vi "UPDATE_volume_by_path.vi"(8 "error in (no error)":errorcluster, 11 "volume path":path) -> (0 "error out":errorcluster)   [LabVIEW 2024]
uses:
  <vilib>/addons/_JKI.lib/Serialization/JSON/JKI JSON Serialization.lvlib
panel:
  in  "from id?":bool
  in  "id":i32
  out "json filename":string
  out "Numeric":i32
  out "appended path":path
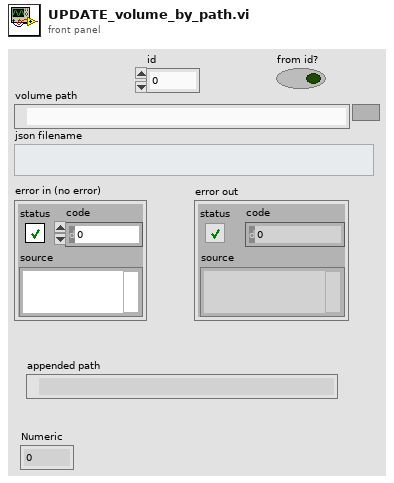
[diagram p1: front panel]
types:
  T1 = typedef "local_volume.ctl" = cluster{"id":i32, "name":string, "sortable_name":string, "aliases":string[], "description":string, "site_detail_url":string, "count_of_issues":i32, "start_year":i32, "publisher_id":i32, "issue_ids":i32[], "date_last_updated":timestamp, "volume":i32, "cv_id":string}
  T2 = typedef "local_issue.ctl" = cluster{"cover_date":timestamp, "id":i32, "cv_id":string, "name":string, "sortable_name":string, "issue_number":string, "deck":string, "description":string, "volume":T3, "store_date":timestamp, "date_last_updated":timestamp, "site_detail_url":string, "cover_url":string, "associated_images":T4[], "characters":T3[], "concepts":T3[], "creators":T5[], "storyArcs":T3[], "teams":T3[]}
  T3 = typedef "comicvine_issue.generic_credit.ctl" = cluster{"id":i32, "name":string}
  T4 = typedef "comicvine_issue.associated_image.ctl" = cluster{"original_url":string, "id":i32}
  T5 = typedef "comicvine_issue.person_credit.ctl" = cluster{"id":i32, "name":string, "role":string}
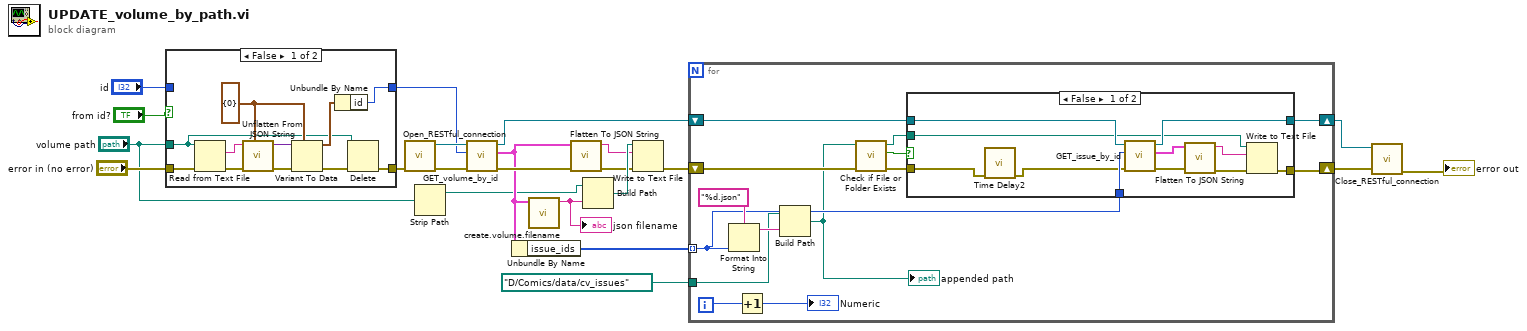
[diagram p0: block diagram]
diagram:
  n1 = case shown="False" "from id?" {
    tunnel: "error in (no error)" -> [w31 w34]
    tunnel: [w27 w34] -> w6
    tunnel: "volume path" -> [w24 _]
    tunnel: [w23 w35] -> w1
    tunnel: "id" -> [_ w35]
    frame False {
      w26 = cluster{"id":i32} {"id"=0}
      n2 = Read from Text File(file (use dialog)=w24, error in=w31) -> (text=w33:string, error out=w30:errorcluster)  [unwired: 2 in, 2 out]
      n3 = call <vilib>:"Unflatten From JSON String.vi"("Type and Defaults"=w26, "error in (no error)"=w30, "JSON String"=w33) -> ("error out"=w29:errorcluster, "Variant"=w32:variant)  [unwired: 7 in]
      n4 = Variant To Data(error in=w29, type=w26, Variant=w32) -> (data=w25:cluster{"id":i32}, error out=w28:errorcluster)
      n5 = Unbundle By Name(w25) -> ("id"=w23:i32)
      n6 = Delete(path (use dialog)=w24, error in=w28) -> (error out=w27:errorcluster)  [unwired: 3 in, 2 out]
    }
    frame True {
    }
  }
  n7 = call "Open_RESTful_connection.vi"("error in (no error)"=w6) -> ("error out"=w12:errorcluster, "REST Client out"=w22:refnum<class "REST Client.lvclass">)  [unwired: 9 in]
  n8 = Strip Path(path="volume path") -> (stripped path=w4:path)  [unwired: 1 out]
  n9 = call "GET_volume_by_id.vi"("error in (no error)"=w12, "volume id"=w1, "REST Client in"=w22) -> ("error out"=w20:errorcluster, "local volume"=w17:T1, "REST Client out"=w16:refnum<class "REST Client.lvclass">)  [unwired: 6 in]
  n10 = Unbundle By Name(w17) -> ("issue_ids"=w15:i32[])
  n11 = call "create.volume.filename.vi"("volume"=w17) -> ("json filename"=w11:string)  [unwired: 10 in]
  "json filename" <- w11
  n12 = call <vilib>:"Flatten To JSON String.vi"("error in (no error)"=w20, "Variant"=w17) -> ("error out"=w18:errorcluster, "JSON String"=w19:string)  [unwired: 8 in]
  n13 = Build Path(base path=w4, name or relative path=w11) -> (appended path=w21:path)
  n14 = Write to Text File(file (use dialog)=w21, text=w19, error in=w18) -> (error out=w13:errorcluster)  [unwired: 1 in, 2 out]
  n15 = for {
    shift-right: [w45] -> w8
    shift-left: w16 -> [w46]
    tunnel: w15 -> [w44] mode=indexing
    tunnel: path "D:/Comics/data/cv_issues" -> [w47]
    shift-right: [w43] -> w10
    shift-left: w13 -> [w42]
    i -> [w41]
    n16 = Format Into String(format string="%d.json", w44) -> (resulting string=w48:string)  [unwired: 2 in, 1 out]
    n17 = Increment(x=w41) -> (x+1=→"Numeric":i32)
    n18 = Build Path(base path=w47, name or relative path=w48) -> (appended path=w38:path)
    "appended path" <- w38
    n19 = call <vilib>:"Check if File or Folder Exists.vi"("error in (no error)"=w42, "path"=w38) -> ("error out"=w39:errorcluster, "file or folder exists?"=w37:bool, "dup path"=w36:path)  [unwired: 7 in]
    n20 = case shown="False" w37 {
      tunnel: w46 -> [w60 w62]
      tunnel: [w59 w62] -> w45
      tunnel: w44 -> [w58 _]
      tunnel: [w53 w61] -> w43
      tunnel: w39 -> [w51 w61]
      tunnel: w36 -> [w52 _]
      frame False {
        n21 = call "Time Delay2"("error in (no error)"=w51) -> ("error out"=w50:errorcluster)  [unwired: 10 in]
        n22 = call "GET_issue_by_id.vi"("error in (no error)"=w50, "issue id"=w58, "REST Client in"=w60) -> ("error out"=w56:errorcluster, "local_issue"=w55:T2, "REST Client out"=w59:refnum<class "REST Client.lvclass">)  [unwired: 6 in]
        n23 = call <vilib>:"Flatten To JSON String.vi"("error in (no error)"=w56, "Variant"=w55) -> ("error out"=w54:errorcluster, "JSON String"=w57:string)  [unwired: 8 in]
        n24 = Write to Text File(file (use dialog)=w52, text=w57, error in=w54) -> (error out=w53:errorcluster)  [unwired: 1 in, 2 out]
      }
      frame True {
      }
    }
  }
  n25 = call "Close_RESTful_connection.vi"("error in (no error)"=w10, "REST Client in"=w8) -> ("error out"=→"error out":errorcluster)  [unwired: 9 in]
